vi "Run Bfr Rx - PingPong - Change Buffer.vi"(7 "Buffer_A":u64 format="%016x", 8 "error in (no error)":errorcluster, 11 "Ping Pong Buffer in":T1 {"Active Buffer Ref" format="%016x"}) -> (0 "error out":errorcluster, 3 "Ping Pong Buffer out":T1 {"Active Buffer Ref" format="%016x"})   [LabVIEW 2016, in "UDP-Custom-Device Engine.lvlib"]
uses:
  UDP-Custom-Device Engine.lvlib
  Types/Engine - Buffered Rx Ping Pong Buffer.ctl
  Types/Engine - Buffered Rx Active Buffer.ctl
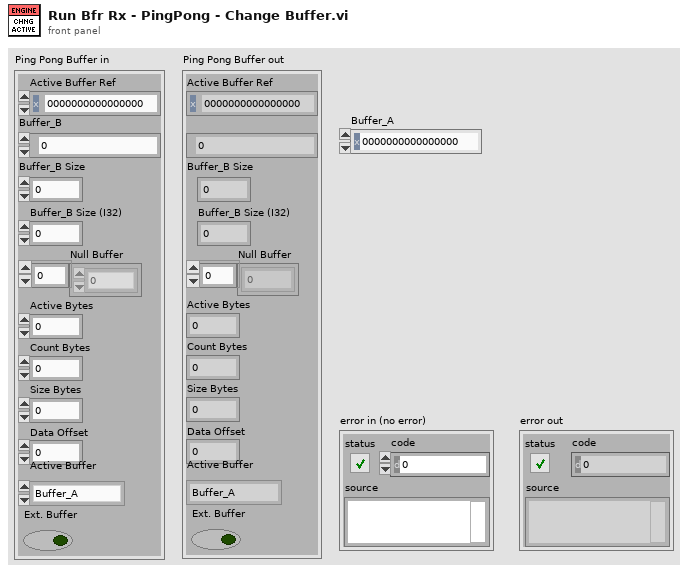
[diagram p1: front panel]
types:
  T1 = typedef "UDP-Custom-Device Engine.lvlib/Engine - Buffered Rx Ping Pong Buffer.ctl" = cluster{"Active Buffer Ref":u64, "Buffer_B":u64, "Buffer_B Size":u64, "Buffer_B Size (I32)":i32, "Null Buffer":u8[], "Active Bytes":u64, "Count Bytes":u64, "Size Bytes":u64, "Data Offset":u64, "Active Buffer":T2, "Ext. Buffer":bool}
  T2 = typedef "UDP-Custom-Device Engine.lvlib/Engine - Buffered Rx Active Buffer.ctl" = enum16{"Buffer_A", "Buffer_B"}
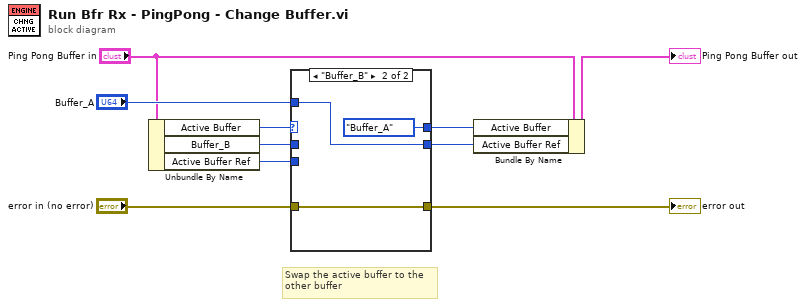
[diagram p0: block diagram]
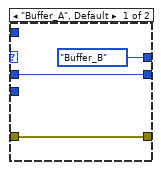
[diagram p2: hidden frame]
diagram:
  # "Swap the active buffer to the\nother buffer"
  n1 = Unbundle By Name("Ping Pong Buffer in") -> ("Active Buffer"=w10:T2, "Buffer_B"=w9:u64, "Active Buffer Ref"=w2:u64)
  n2 = case shown="\"Buffer_B\"" w10 {
    tunnel: w9 -> [w12 _]
    tunnel: "Buffer_A" -> [_ w16]
    tunnel: [w13 w15] -> w7
    tunnel: "error in (no error)" -> [w13 w15]
    tunnel: [w12 w16] -> w6
    tunnel: w2 -> [_ _]
    tunnel: [Engine_-_Buffered_Rx_Active_Buffer."Buffer_B" ("Active Buffer") Engine_-_Buffered_Rx_Active_Buffer."Buffer_A" ("Active Buffer")] -> w1
    frame "Buffer_A", Default {
    }
    frame "Buffer_B" {
    }
  }
  "error out" <- w7
  n3 = Bundle By Name(cluster="Ping Pong Buffer in", "Active Buffer"=w1, "Active Buffer Ref"=w6) -> (→"Ping Pong Buffer out":T1)
